vi "QMH_Handle_LED.vi"() -> ()   [LabVIEW 2015]
uses:
  <vilib>/ErrorRing/Error Ring.xnode
panel:
  in  "Event Fired! 2":refnum<vi>
  out "x-y":i32(slide) scale=0.0..100.0
  out "Boolean":bool
  out "Numeric Indicator":i16
  in  "Blank Button":bool caption="Fire Event"
  in  "stop":bool
  out "Event Fired!":bool
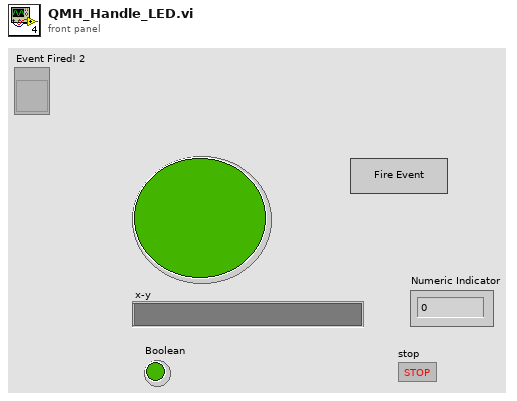
[diagram p1: front panel]
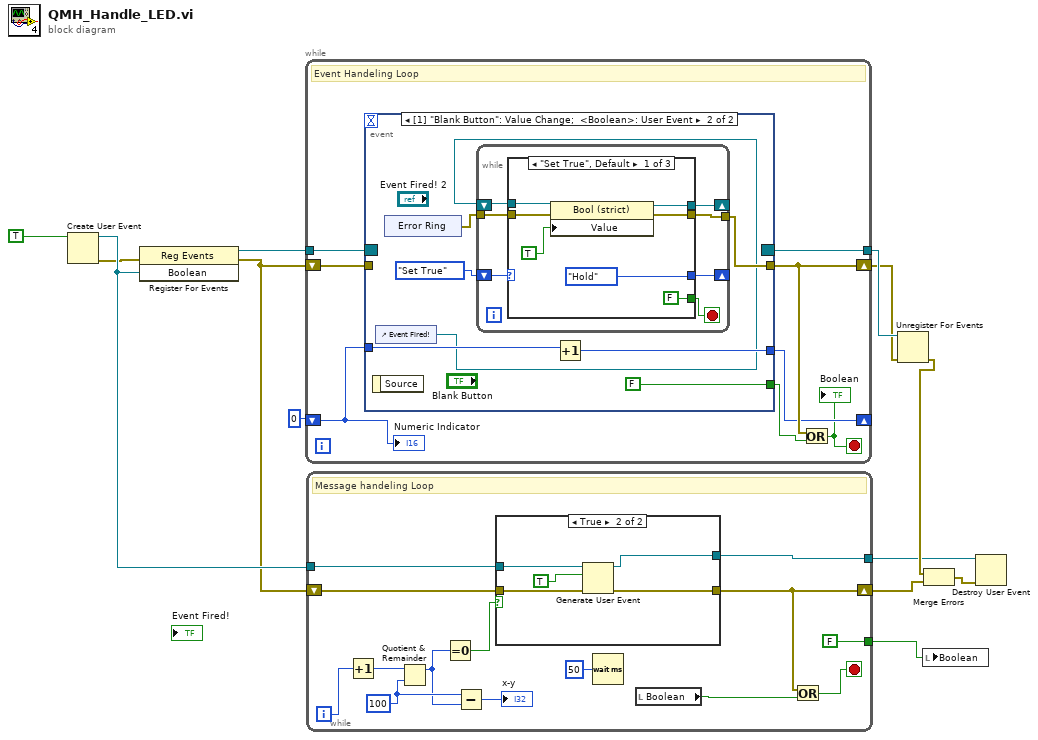
[diagram p0: block diagram]
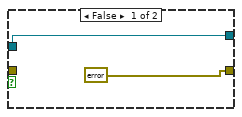
[diagram p2: hidden frame]
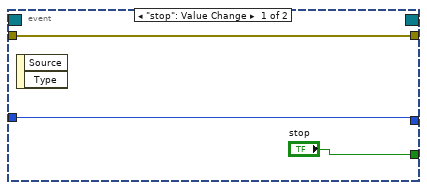
[diagram p3: hidden frame]
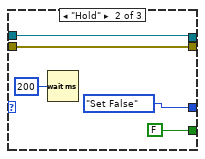
[diagram p4: hidden frame]
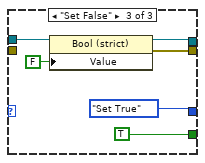
[diagram p5: hidden frame]
diagram:
  n1 = Create User Event(user event datatype=TRUE ("Boolean")) -> (user event=w9:refnum<user-event>, error out=w8:errorcluster)  [unwired: 1 in]
  n2 = register-events(error in=w8, w9) -> (reference out=w12:refnum<event-registration>, error out=w3:errorcluster)  [unwired: 1 in]
  n3 = while {
    tunnel: [w21] -> w13
    tunnel: w12 -> [w20]
    shift-right: [w15] -> _
    shift-left: i16 0 -> [w16]
    shift-right: [w18] -> w11
    shift-left: w3 -> [w19]
    stop <- w14 stop-if-true
    # "Event Handeling Loop"
    n4 = event shown="[1] \"Blank Button\": Value Change;  <Boolean>: User Event" {
      selector: w20 -> [_ _]
      dyn-events: [_ _] -> w21
      timeout: _ -> [_ _]
      tunnel: w19 -> [w24 _]
      tunnel: [w24 w27] -> w18
      tunnel: ["stop" FALSE] -> w17
      tunnel: w16 -> [w22 w30]
      tunnel: [w22 w29] -> w15
      event "stop": Value Change {
        n5 = event-data() -> ()  [unwired: 1 in, 2 out]
      }
      event "Blank Button": Value Change; User Event {
        n6 = event-data() -> ()  [unwired: 1 in, 1 out]
        n7 = control-ref of="Event Fired!"() -> (w26:refnum<vi>)
        n8 = xnode "Error Ring"() -> ("error out"=w28:errorcluster)
        n9 = while {
          tunnel: w28 -> [w38]
          shift-right: [w36] -> _
          shift-left: w26 -> [w39]
          tunnel: [w35] -> w27
          shift-right: [w33] -> _
          shift-left: enum16{"Hold", "Set True", "Set False"}."Set True" -> [w34]
          stop <- w37 stop-if-true
          n10 = case shown="\"Set True\", Default" w34 {
            tunnel: w39 -> [w46 w51 w57]
            tunnel: w38 -> [w45 w50 _]
            tunnel: [FALSE FALSE TRUE] -> w37
            tunnel: [w44 w50 w53] -> w35
            tunnel: [w43 w51 w54] -> w36
            tunnel: [enum16{"Hold", "Set True", "Set False"}."Hold" enum16{"Hold", "Set True", "Set False"}."Set False" enum16{"Hold", "Set True", "Set False"}."Set True"] -> w33
            frame "Set True", Default {
              n11 = property class="Bool (strict)"(reference=w46, error in=w45, "Value"=TRUE) -> (reference out=w43:refnum<vi>, error out=w44:errorcluster)
            }
            frame "Hold" {
              n12 = Wait (ms)(milliseconds to wait=u32 200) -> ()  [unwired: 1 out]
            }
            frame "Set False" {
              n13 = property class="Bool (strict)"(reference=w57, "Value"=FALSE) -> (reference out=w54:refnum<vi>, error out=w53:errorcluster)  [unwired: 1 in]
            }
          }
        }
        n14 = Increment(x=w30) -> (x+1=w29:i16)
      }
    }
    n15 = Or(x=w18, y=w17) -> (x .or. y?=w14:bool)
    "Boolean" <- w14
    "Numeric Indicator" <- w16
  }
  n16 = while {
    tunnel: w9 -> [w71]
    tunnel: [w70] -> w4
    shift-right: [w68] -> w7
    shift-left: w3 -> [w67]
    tunnel: [FALSE] -> w1
    i -> [w65]
    stop <- w69 stop-if-true
    w62 = 100
    # "Message handeling Loop"
    n17 = Increment(x=w65) -> (x+1=w64:i32)
    n18 = Quotient & Remainder(x=w64, y=w62) -> (x-y*floor(x/y)=w61:i32)  [unwired: 1 out]
    n19 = Equal To 0?(x=w61) -> (x = 0?=w63:bool)
    n20 = Subtract(x=w62, y=w61) -> (x-y=→"x-y":i32)
    n21 = case shown="True" w63 {
      tunnel: w71 -> [w72 w78]
      tunnel: w67 -> [_ w77]
      tunnel: [errorcluster {"status"=FALSE, "code"=0, "source"=""} ("error constant") w76] -> w68
      tunnel: [w72 w75] -> w70
      frame False {
      }
      frame True {
        n22 = Generate User Event(user event=w78, event data cluster=TRUE, error in=w77) -> (user event out=w75:refnum<user-event>, error out=w76:errorcluster)  [unwired: 1 in]
      }
    }
    n23 = Wait (ms)(milliseconds to wait=u32 50) -> ()  [unwired: 1 out]
    n24 = local read "Boolean"() -> (w66:bool)
    n25 = Or(x=w68, y=w66) -> (x .or. y?=w69:bool)
  }
  n26 = Unregister For Events(event registration refnum=w13, error in=w11) -> (error out=w6:errorcluster)
  n27 = local write "Boolean"(w1) -> ()
  n28 = Merge Errors(w6, w7) -> (w5:errorcluster)
  n29 = Destroy User Event(user event=w4, error in=w5) -> ()  [unwired: 1 out]
